vi "Send Async Message.vi"(5 "Component ID":u8, 7 "FPGA Interface":refnum<class "FPGA Interface.lvclass">, 8 "error in (no error)":errorcluster, 10 "Async Message":refnum<class "Async Message.lvclass">, 11 "Bus Controller in":refnum<class "Bus Controller.lvclass">) -> (0 "error out":errorcluster, 3 "Bus Controller out":refnum<class "Bus Controller.lvclass">)   [LabVIEW 2020, in "BCI-1553 API.lvlib" / "Bus Controller.lvclass"]
doc: "Sends an Asynchronous Message out on this Bus Controller. The Bus Controller must be started already before an Asynchronous Message can be sent."
uses:
  Bus Controller.lvclass
  C:/Users/MattJ/Desktop/git/bci-1553-labview-api/src/1553 SubComponent/1553 SubComponent.lvclass
  Frames & Messages/Async Message/Async Message.lvclass
  Dependencies/FPGA Interface/FPGA Interface.lvclass
  Bus Controller.lvclass/Bus Controller.ctl
  Dependencies/Registry/Registry.lvclass
panel:
  in  "Trig":u16=4 format="%04x"
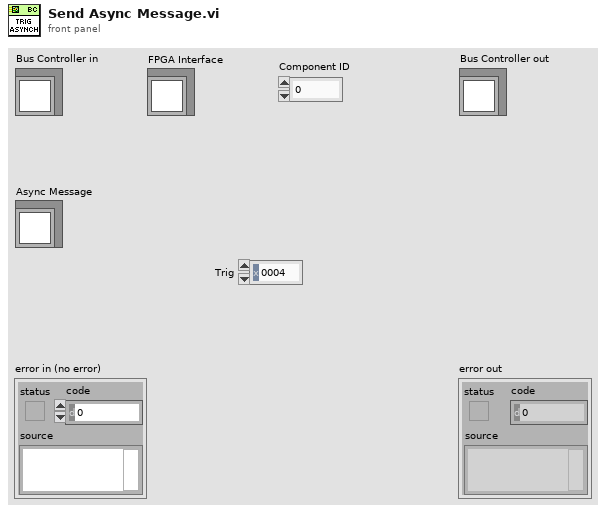
[diagram p1: front panel]
types:
  T1 = typedef "BCI-1553 API.lvlib/Async Message Pointers.ctl" = cluster{"HP Async Control Addresses":u16[], "HP Async Data Addresses":u16[], "LP Async Control Addresses":u16[], "LP Async Data Addresses":u16[]}
  T2 = typedef "BCI-1553 API.lvlib/Async Payload.ctl" = cluster{"Configuration Address":u16, "Configuration":u16[], "Data Address":u16, "Data":u16[], "Trigger Command":u16, "Command Type":enum16{"Transmit", "Receive"}}
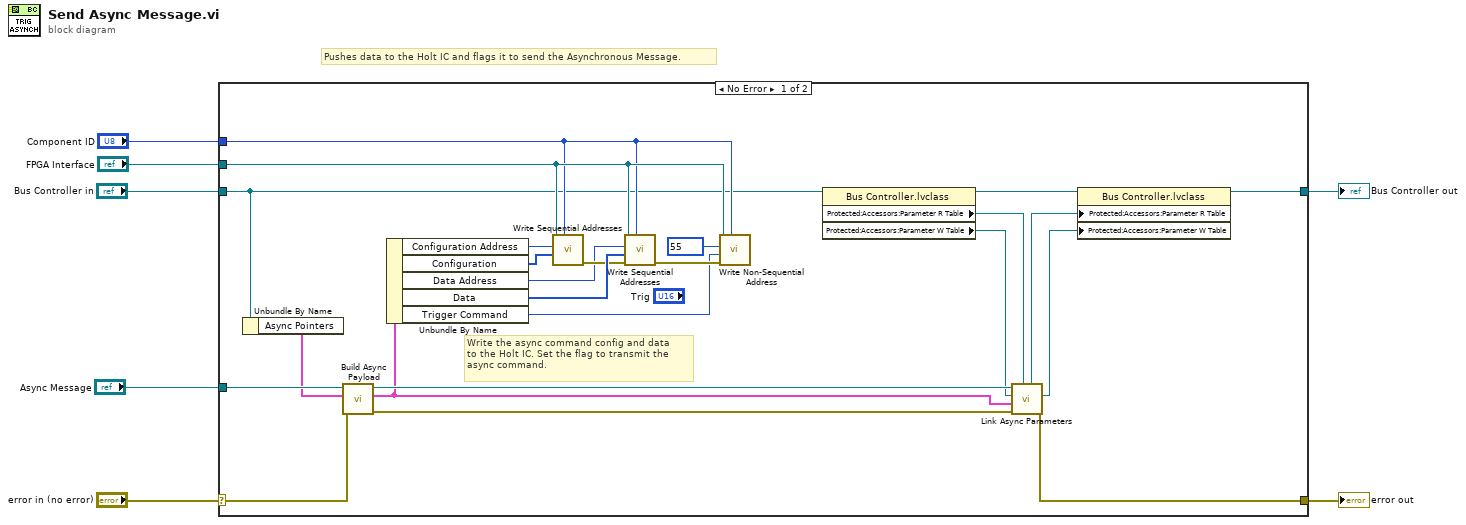
[diagram p0: block diagram]
diagram:
  # "Pushes data to the Holt IC and flags it to send the Asynchronous Message."
  n1 = case shown="No Error" "error in (no error)" {
    selector: "error in (no error)" -> [w29 w33]
    tunnel: [w15 w33] -> w6
    tunnel: [w18 w32] -> w4
    tunnel: "Bus Controller in" -> [w19 w32]
    tunnel: "Async Message" -> [w31 _]
    tunnel: "FPGA Interface" -> [w24 _]
    tunnel: "Component ID" -> [w23 _]
    frame No Error {
      # "Write the async command config and data\nto the Holt IC. Set the flag to transmit the\nasync command."
      n2 = Unbundle By Name(w19) -> ("Async Pointers"=w30:T1)
      n3 = call-dynamic "Build Async Payload.vi"("error in (no error)"=w29, "Async Pointers"=w30, "Async Message in"=w31) -> ("error out"=w16:errorcluster, "Async Payload"=w14:T2, "Async Message out"=w17:refnum<class "Async Message.lvclass">)  [unwired: 6 in]
      n4 = Unbundle By Name(w14) -> ("Configuration Address"=w28:u16, "Configuration"=w27:u16[], "Data Address"=w9:u16, "Data"=w26:u16[], "Trigger Command"=w8:u16)
      n5 = call-dynamic "Write Sequential Addresses.vi"("Target IC (1-8)"=w23, "Data"=w27, "Starting Address"=w28, "FPGA Interface in"=w24) -> ("error out"=w25:errorcluster)  [unwired: 7 in]
      n6 = call-dynamic "Write Sequential Addresses.vi"("Target IC (1-8)"=w23, "error in (no error)"=w25, "Data"=w26, "Starting Address"=w9, "FPGA Interface in"=w24) -> ("error out"=w22:errorcluster)  [unwired: 6 in]
      n7 = call-dynamic "Write Non-Sequential Address.vi"("Target IC (1-8)"=w23, "error in (no error)"=w22, "Data"=w8, "Address"=u16 55 ("Command Word"), "FPGA Interface in"=w24) -> ()  [unwired: 6 in, 1 out]
      n8 = property class="Bus Controller.lvclass"(reference=w19) -> (reference out=w20:refnum<class "Bus Controller.lvclass">, "Protected:Accessors:Parameter R Table"=w11:refnum<class "Registry.lvclass">, "Protected:Accessors:Parameter W Table"=w12:refnum<class "Registry.lvclass">)  [unwired: 1 in, 1 out]
      n9 = call-dynamic "Link Async Parameters.vi"("Parameter R Table"=w11, "error in (no error)"=w16, "Async Payload"=w14, "Parameter W Table"=w12, "Async Message in"=w17) -> ("error out"=w15:errorcluster, "Parameter W Table out"=w13:refnum<class "Registry.lvclass">, "Parameter R Table out"=w10:refnum<class "Registry.lvclass">)  [unwired: 3 in, 1 out]
      n10 = property class="Bus Controller.lvclass"(reference=w20, "Protected:Accessors:Parameter R Table"=w10, "Protected:Accessors:Parameter W Table"=w13) -> (reference out=w18:refnum<class "Bus Controller.lvclass">)  [unwired: 1 in, 1 out]
    }
    frame Error {
    }
  }
  "error out" <- w6
  "Bus Controller out" <- w4
